vi "DaxSelection.vi"(11 "Daxsonics Present":refnum<visa-resource-name>[](array[refnum])) -> (0 "Daxsonics Name":T1, 3 "Selected Daxsonics":refnum<visa-resource-name>)   [LabVIEW 2022 SP3]
uses:
  Daxsonics_Pulsers.ctl
  PulserGlobals.vi
panel:
  in  "New2021":bool
  in  "10ERS8":bool
  in  "BP1":bool
  in  "BP2B":bool
  in  "BP2A":bool
  # "Multiple Daxsonics Detected, Please Choose 1"
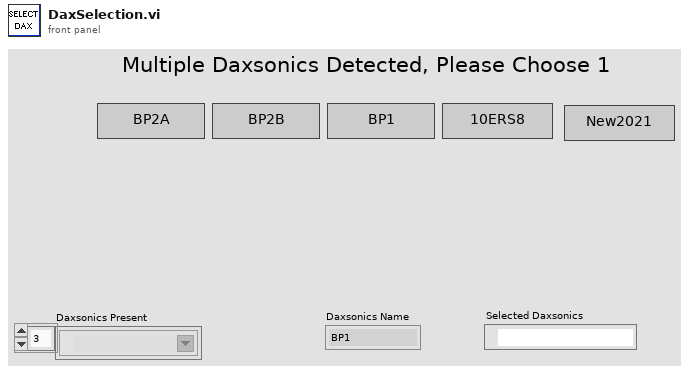
[diagram p1: front panel]
types:
  T1 = typedef "Daxsonics_Pulsers.ctl" = enum16{"BP1", "BP2_A", "BP2_B", "10ERS8", "New2021"}
  T2 = enum8{"Enabled", "Disabled", "Disabled and Grayed Out"}
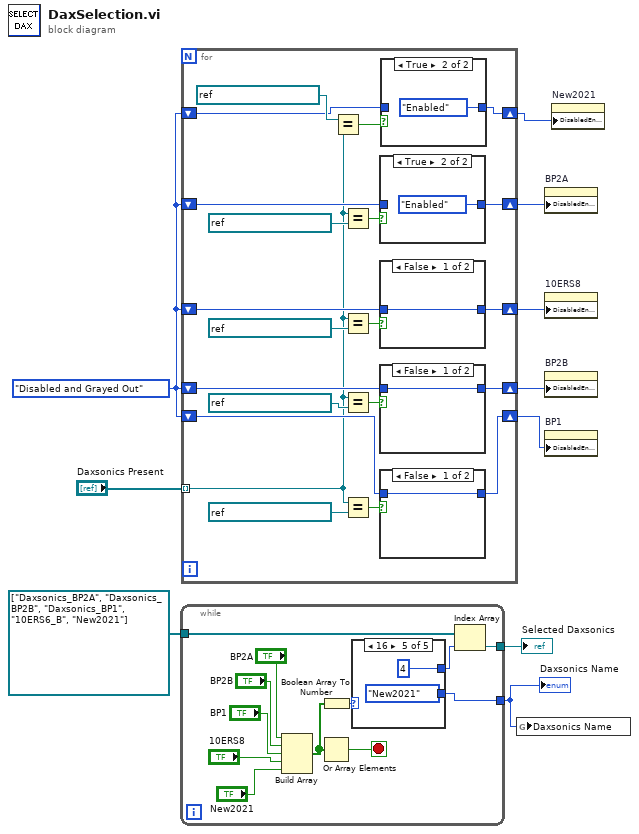
[diagram p0: block diagram]
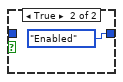
[diagram p3: hidden frame]
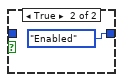
[diagram p4: hidden frame]
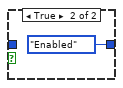
[diagram p5: hidden frame]
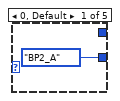
[diagram p7: hidden frame]
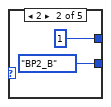
[diagram p8: hidden frame]
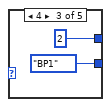
[diagram p9: hidden frame]
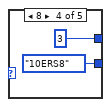
[diagram p10: hidden frame]
diagram:
  w2 = T2."Disabled and Grayed Out" ("Disabled")
  n1 = while {
    tunnel: refnum<visa-resource-name>[] ["Daxsonics_BP2A", "Daxsonics_BP2B", "Daxsonics_BP1", "10ERS6_B", "New2021"] -> [w15]
    tunnel: [w14] -> w10
    tunnel: [w12] -> w3
    stop <- w18 stop-if-true
    n2 = Build Array("BP2A", "BP2B", "BP1", "10ERS8", "New2021") -> (w17:bool[])
    n3 = Or Array Elements(Boolean array=w17) -> (logical OR=w18:bool)
    n4 = Boolean Array To Number(Boolean array=w17) -> (number=w16:u32)
    n5 = case shown="16" w16 {
      tunnel: [_ 1 2 3 4] -> w13
      tunnel: [Daxsonics_Pulsers."BP2_A" ("Daxsonics Name") Daxsonics_Pulsers."BP2_B" ("Daxsonics Name") Daxsonics_Pulsers."BP1" ("Daxsonics Name") Daxsonics_Pulsers."10ERS8" ("Daxsonics Name") Daxsonics_Pulsers."New2021" ("Daxsonics Name")] -> w12
      frame 0, Default {
      }
      frame 2 {
      }
      frame 4 {
      }
      frame 8 {
      }
      frame 16 {
      }
    }
    n6 = Index Array(array=w15, index=w13) -> (element=w14:refnum<visa-resource-name>)
  }
  "Selected Daxsonics" <- w10
  "Daxsonics Name" <- w3
  n7 = for {
    tunnel: "Daxsonics Present" -> [w34] mode=indexing
    shift-right: [w41] -> w5
    shift-left: w2 -> [w38]
    shift-right: [w40] -> w4
    shift-left: w2 -> [w37]
    shift-right: [w42] -> w6
    shift-left: w2 -> [w39]
    shift-right: [w47] -> w7
    shift-left: w2 -> [w46]
    shift-right: [w32] -> w1
    shift-left: w2 -> [w33]
    n8 = Equal?(x=refnum<visa-resource-name> "Dax2021" ("VISA resource name"), y=w34) -> (x = y?=w35:bool)
    n9 = Equal?(x=w34, y=refnum<visa-resource-name> "Daxsonics_BP2A" ("VISA resource name")) -> (x = y?=w48:bool)
    n10 = Equal?(x=w34, y=refnum<visa-resource-name> "10ERS8" ("VISA resource name")) -> (x = y?=w45:bool)
    n11 = Equal?(x=w34, y=refnum<visa-resource-name> "Daxsonics_BP2B" ("VISA resource name")) -> (x = y?=w44:bool)
    n12 = Equal?(x=w34, y=refnum<visa-resource-name> "Daxsonics_BP1" ("VISA resource name")) -> (x = y?=w43:bool)
    n13 = case shown="True" w48 {
      tunnel: [w61 T2."Enabled" ("Disabled")] -> w47
      tunnel: w46 -> [w61 _]
      frame False {
      }
      frame True {
      }
    }
    n14 = case shown="False" w45 {
      tunnel: [w59 T2."Enabled" ("Disabled")] -> w42
      tunnel: w39 -> [w59 _]
      frame False {
      }
      frame True {
      }
    }
    n15 = case shown="False" w44 {
      tunnel: [w57 T2."Enabled" ("Disabled")] -> w41
      tunnel: w38 -> [w57 _]
      frame False {
      }
      frame True {
      }
    }
    n16 = case shown="False" w43 {
      tunnel: [w55 T2."Enabled" ("Disabled")] -> w40
      tunnel: w37 -> [w55 _]
      frame False {
      }
      frame True {
      }
    }
    n17 = case shown="True" w35 {
      tunnel: [w53 T2."Enabled" ("Disabled")] -> w32
      tunnel: w33 -> [w53 _]
      frame False {
      }
      frame True {
      }
    }
  }
  n18 = global write "PulserGlobals.vi" "Daxsonics Name"(w3) -> ()
  n19 = property on="BP2A" class="Bool"("DisabledEnum"=w7) -> ()  [unwired: 2 in, 2 out]
  n20 = property on="10ERS8" class="Bool"("DisabledEnum"=w6) -> ()  [unwired: 2 in, 2 out]
  n21 = property on="BP2B" class="Bool"("DisabledEnum"=w5) -> ()  [unwired: 2 in, 2 out]
  n22 = property on="BP1" class="Bool"("DisabledEnum"=w4) -> ()  [unwired: 2 in, 2 out]
  n23 = property on="New2021" class="Bool"("DisabledEnum"=w1) -> ()  [unwired: 2 in, 2 out]
